vi "accept.vi"(0 "HGF_Visitable":refnum<class "HGF_Visitable.lvclass">, 2 "HGF_Visitor":refnum<class "HGF_Visitor.lvclass">, 5 "error in (no error)":errorcluster) -> (14 "dup HGF_Visitable":refnum<class "HGF_Visitable.lvclass">, 16 "dup HGF_Visitor":refnum<class "HGF_Visitor.lvclass">, 19 "error out":errorcluster)   [LabVIEW 2014, in "HGF_BaseClasses.lvlib" / "HGF_Visitable.lvclass"]
doc: "This is a static VI that calls Visitor.visit() to perform the Visitor.action() which means: calling public methods of Visitable child class.\n\n<B>Attention:</B> The Visitor is accepted if its addressee is an empty string or equals the Visitable's objectName."
uses:
  HGF_Visitable.lvclass
  HGF_Visitor/HGF_Visitor.lvclass
  HGF_Auxiliary/HGF_Auxiliary.lvlib
  HGF_Auxiliary/Severity.ctl
  HGF_Auxiliary/ErrorCode.ctl
  HGF_Factory/HGF_Factory.lvclass
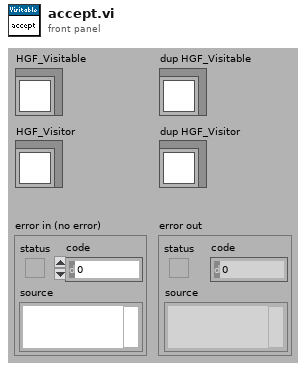
[diagram p1: front panel]
types:
  T1 = typedef "HGF_Auxiliary.lvlib/ErrorCode.ctl" = enum32{"No error", "Function not supported.", "This VI is for friends only.", "Reference object aready exisits.", "Parameter out of range.", "Not a rendezvous.", "Invalid notifier reference.", "Invalid queue reference.", "Self-Test not supported.", "Reset not supported.", "IDN query not supported.", "Error query not supported.", "Incorrect addressee.", "Object already exists.", "No class name specified", "Driver not supported", "Attribute is not writable"}
  T2 = typedef "HGF_Auxiliary.lvlib/Severity.ctl" = enum16{"Info", "Warning", "Fault", "Error", "Fatal"}
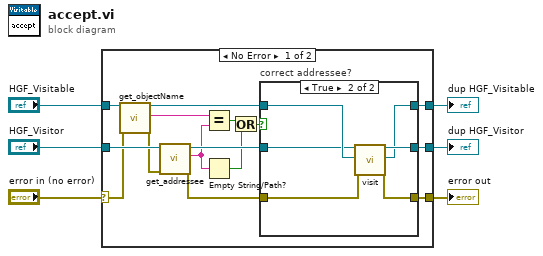
[diagram p0: block diagram]
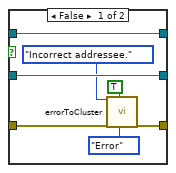
[diagram p2: hidden frame]
diagram:
  n1 = case shown="No Error" "error in (no error)" {
    selector: "error in (no error)" -> [w9 w37]
    tunnel: [w20 w37] -> w5
    tunnel: [w19 w36] -> w3
    tunnel: "HGF_Visitable" -> [w18 w36]
    tunnel: "HGF_Visitor" -> [w16 w35]
    tunnel: [w21 w35] -> w1
    frame No Error {
      n2 = call "get_objectName.vi"("HGF_Factory"=w18, "error in (no error)"=w9) -> ("dup HGF_Factory"=w17:refnum<class "HGF_Visitable.lvclass">, "objectName"=w14:string, "error out"=w8:errorcluster)  [unwired: 15 out]
      n3 = call "get_addressee.vi"("error in (no error)"=w8, "HGF_Visitor"=w16) -> ("error out"=w7:errorcluster, "addressee"=w13:string, "dup HGF_Visitor"=w15:refnum<class "HGF_Visitor.lvclass">)  [unwired: 7 out]
      n4 = Equal?(x=w14, y=w13) -> (x = y?=w12:bool)
      n5 = Empty String/Path?(string/path=w13) -> (empty?=w11:bool)
      n6 = Or(x=w12, y=w11) -> (x .or. y?=w10:bool)
      n7 = case "correct addressee?" shown="True" w10 {
        tunnel: [w27 w34] -> w21
        tunnel: [w25 w33] -> w20
        tunnel: [w28 w32] -> w19
        tunnel: w17 -> [w28 w31]
        tunnel: w15 -> [w27 w30]
        tunnel: w7 -> [w26 w29]
        frame False {
          n8 = call "errorToCluster.vi"("error code"=ErrorCode."Incorrect addressee.", "error in (no error)"=w26, "show call chain? (True)"=TRUE, "severity (Error)"=Severity."Error") -> ("error out"=w25:errorcluster)  [unwired: 1 in, 14 out]
        }
        frame True {
          n9 = call "visit.vi"("HGF_Visitor"=w30, "HGF_Visitable"=w31, "error in (no error)"=w29) -> ("dup HGF_Visitor"=w34:refnum<class "HGF_Visitor.lvclass">, "dup HGF_Visitable"=w32:refnum<class "HGF_Visitable.lvclass">, "error out"=w33:errorcluster)  [unwired: 14 out]
        }
      }
    }
    frame Error {
    }
  }
  "error out" <- w5
  "dup HGF_Visitable" <- w3
  "dup HGF_Visitor" <- w1
